vi "Write Alive_.vi"(8 "error in (no error)":errorcluster, 10 "Alive?":bool, 11 "PlayerUpdate in":refnum<class "PlayerUpdate.lvclass">) -> (0 "error out":errorcluster, 3 "PlayerUpdate out":refnum<class "PlayerUpdate.lvclass">)   [LabVIEW 2019, in "PlayerUpdate.lvclass"]
uses:
  PlayerUpdate.lvclass
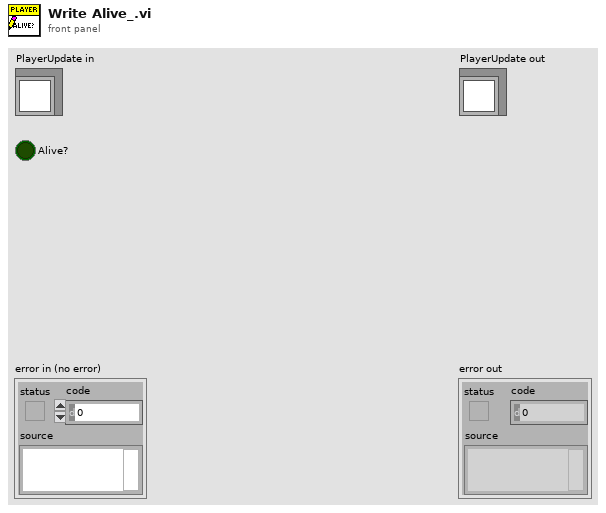
[diagram p1: front panel]
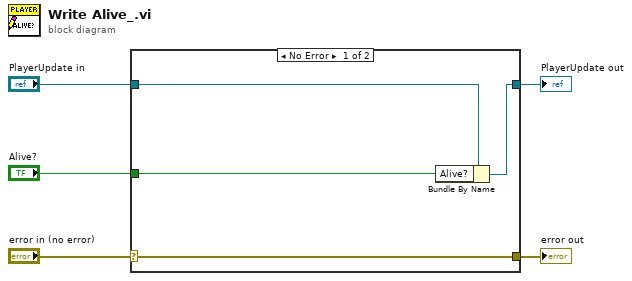
[diagram p0: block diagram]
diagram:
  n1 = case shown="No Error" "error in (no error)" {
    selector: "error in (no error)" -> [w9 w10]
    tunnel: [w9 w10] -> w4
    tunnel: [w7 w11] -> w2
    tunnel: "PlayerUpdate in" -> [w8 w11]
    tunnel: "Alive?" -> [w6 _]
    frame No Error {
      n2 = Bundle By Name(cluster=w8, "Alive?"=w6) -> (w7:refnum<class "PlayerUpdate.lvclass">)
    }
    frame Error {
    }
  }
  "error out" <- w4
  "PlayerUpdate out" <- w2
